vi "Get Timeout.vi"(8 "error in (no error)":errorcluster, 11 "ScrollingList in":refnum<class "ScrollingList.lvclass">) -> (0 "error out":errorcluster, 2 "Timeout":i32, 3 "ScrollingList (dup)":refnum<class "ScrollingList.lvclass">)   [LabVIEW 2020, in "ScrollingList.lvclass"]
uses:
  ScrollingList.lvclass
  ScrollingList.lvclass/ScrollingList.ctl
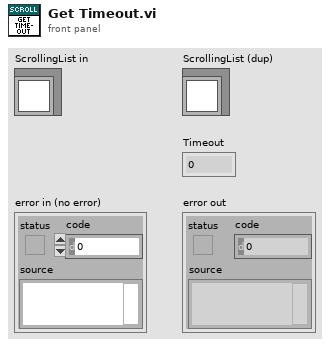
[diagram p1: front panel]
types:
  T1 = typedef "ScrollingList.lvclass/State Data.ctl" = cluster{"Timeout":i32, "Time":timestamp, "Y":i32, "Origin:Top":i16, "Rate":dbl, "ListItems":string[], "Item Height":i32, "Max Height":i32}
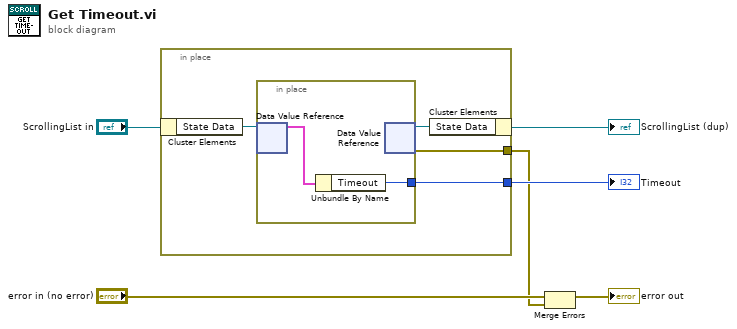
[diagram p0: block diagram]
diagram:
  n1 = in-place {
    in-place-border: [w8] -> w4
    in-place-border: [w7] -> w1
    n2 = in-place-cluster #1("ScrollingList in") -> ("State Data"=w10:refnum<data-value>)
    n3 = in-place {
      in-place-border: [w11] -> w8
      n4 = in-place-dvr #2(w10) -> (w12:T1)  [unwired: 1 out]
      n5 = Unbundle By Name(w12) -> ("Timeout"=w11:i32)
      n6 = in-place-dvr #2() -> (w9:refnum<data-value>, w7:errorcluster)  [unwired: 1 in]
    }
    n7 = in-place-cluster #1("State Data"=w9) -> (→"ScrollingList (dup)":refnum<class "ScrollingList.lvclass">)
  }
  "Timeout" <- w4
  n8 = Merge Errors("error in (no error)", w1) -> (→"error out":errorcluster)
